vi "Buttons Pressed.vi"(1 "Button Values":bool[](array[boolean])) -> (0 "Button Presses":bool[](array[boolean]))   [LabVIEW 2015]
doc: "This VI compares button states to identify when a button is first pressed."
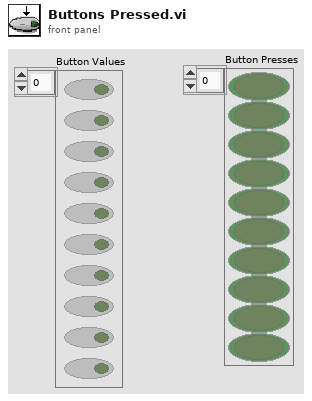
[diagram p1: front panel]
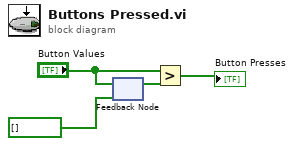
[diagram p0: block diagram]
diagram:
  n1 = feedback #1(bool[] [] ("Button Values")) -> (w4:bool[])
  n2 = feedback-in #1("Button Values") -> ()
  n3 = Greater?(x="Button Values", y=w4) -> (0:→"Button Presses":bool[])
